vi "Frame Update GoTo Index.vi"(8 "error in (no error)":errorcluster, 10 "Frame Num":u32, 11 "LF2R IDE in":refnum<class "Main Panel.lvclass">) -> (0 "error out":errorcluster, 3 "LF2R IDE out":refnum<class "Main Panel.lvclass">)   [LabVIEW 2018, in "Main Panel.lvlib" / "Main Panel.lvclass"]
uses:
  Main Panel.lvclass
  Main Panel.lvclass/Main Panel.ctl
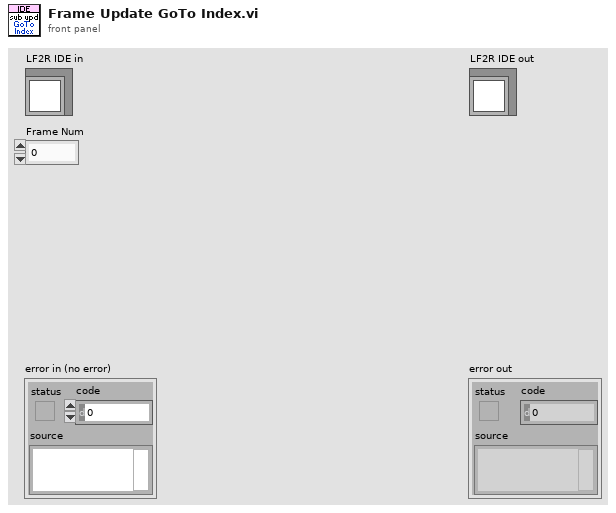
[diagram p1: front panel]
types:
  T1 = typedef "LVStringsAndValuesArrayTypeDef_U16.ctl" = cluster{"String":string, "Value":u16}[]
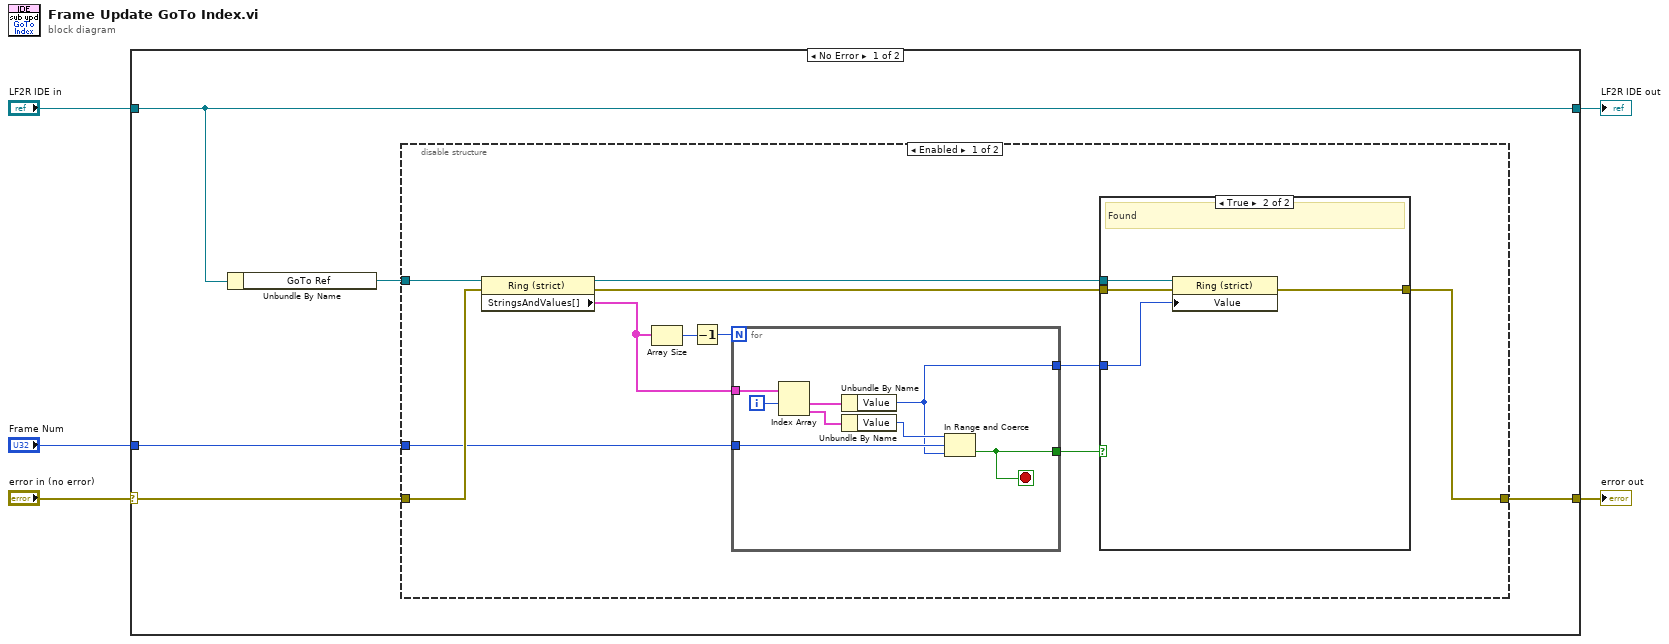
[diagram p0: block diagram]
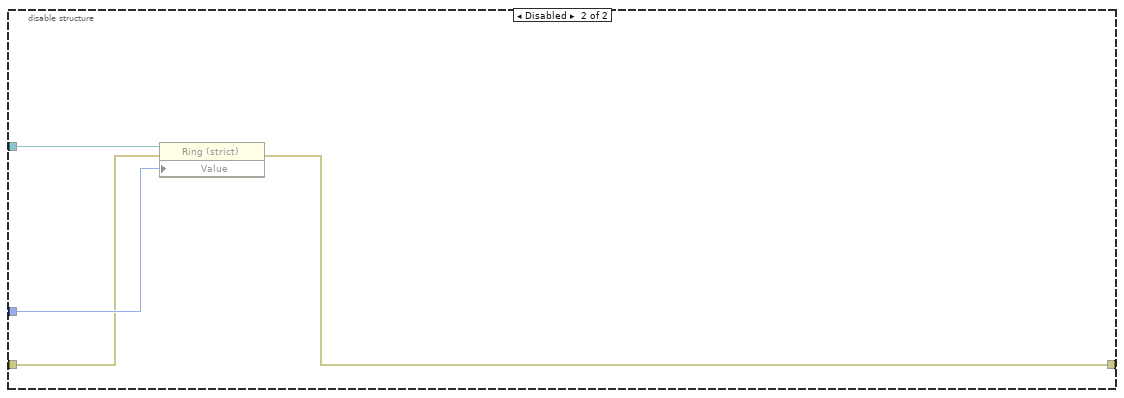
[diagram p3: hidden frame]
diagram:
  n1 = case shown="No Error" "error in (no error)" {
    selector: "error in (no error)" -> [w8 w40]
    tunnel: [w6 w40] -> w4
    tunnel: [w9 w39] -> w2
    tunnel: "LF2R IDE in" -> [w9 w39]
    tunnel: "Frame Num" -> [w7 _]
    frame No Error {
      n2 = Unbundle By Name(w9) -> ("GoTo Ref"=w10:refnum<vi>)
      n3 = disable-structure shown="Enabled" {
        disable-tunnel: w10 -> [w21 w38]
        disable-tunnel: w8 -> [w20 w36]
        disable-tunnel: w7 -> [w16 w37]
        disable-tunnel: [w11 w35] -> w6
        frame Enabled {
          n4 = property class="Ring (strict)"(reference=w21, error in=w20) -> (reference out=w14:refnum<vi>, error out=w12:errorcluster, "StringsAndValues[]"=w17:T1)
          n5 = Array Size(array=w17) -> (size(s)=w19:i32)
          n6 = Decrement(x=w19) -> (x-1=w18:i32)
          n7 = for {
            N: w18 -> [_]
            tunnel: w17 -> [w34]
            tunnel: w16 -> [w30]
            tunnel: [w29] -> w15
            tunnel: [w27] -> w13
            i -> [w28]
            stop <- w29 stop-if-true
            n8 = Index Array(array=w34, index #1=w28) -> (element #1=w33:cluster{"String":string, "Value":u16}, element #2=w32:cluster{"String":string, "Value":u16})  [unwired: 1 in]
            n9 = Unbundle By Name(w33) -> ("Value"=w27:u16)
            n10 = Unbundle By Name(w32) -> ("Value"=w31:u16)
            n11 = In Range and Coerce(upper limit=w31, x=w30, lower limit=w27) -> (In Range?=w29:bool)  [unwired: 1 out]
          }
          n12 = case shown="True" w15 {
            tunnel: w14 -> [_ w26]
            tunnel: w13 -> [_ w25]
            tunnel: w12 -> [w22 w24]
            tunnel: [w22 w23] -> w11
            frame False {
            }
            frame True {
              # "Found"
              n13 = property class="Ring (strict)"(reference=w26, error in=w24, "Value"=w25) -> (error out=w23:errorcluster)  [unwired: 1 out]
            }
          }
        }
        frame Disabled {
          n14 = property class="Ring (strict)"(reference=w38, error in=w36, "Value"=w37) -> (error out=w35:errorcluster)  [unwired: 1 out]
        }
      }
    }
    frame Error {
    }
  }
  "error out" <- w4
  "LF2R IDE out" <- w2
